vi "flow_to_coag_dose.vi"(4 "State":i16, 5 "Time":dbl format="%.2f", 6 "Sensor Values":dbl[](array[numeric]), 7 "Set Points":dbl[](array[numeric])) -> (0 "required data":T1={"Set Point names"=["pump flow (mL/s)", "", ""], "required number of setpoints"=1, "required number of sensors"=1, "Sensor names"=["raw flow rate (L/s)"]}, 3 "output value":dbl)   [LabVIEW 2019]
uses:
  Global Plantita Parameters.vi
panel:
  # "Enter the correct information for this control code in the required data structure below. Then make the current value default by right clicking on the border of the data structure. Select \"data operations\" and then select \"make current value default\". These values will be displayed by process controller."
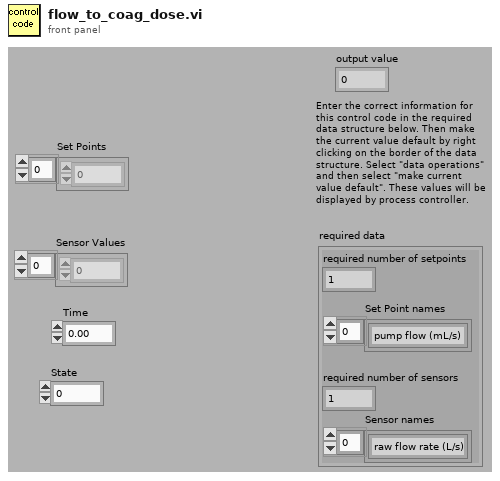
[diagram p1: front panel]
types:
  T1 = cluster{"Set Point names":string[], "required number of setpoints":u8, "required number of sensors":u8, "Sensor names":string[]}
  T2 = cluster{"flocculation_time(s)":dbl, "clarification_time(s)":dbl, "height_ff(m)":dbl, "C_coag_stock(g/L)":dbl}
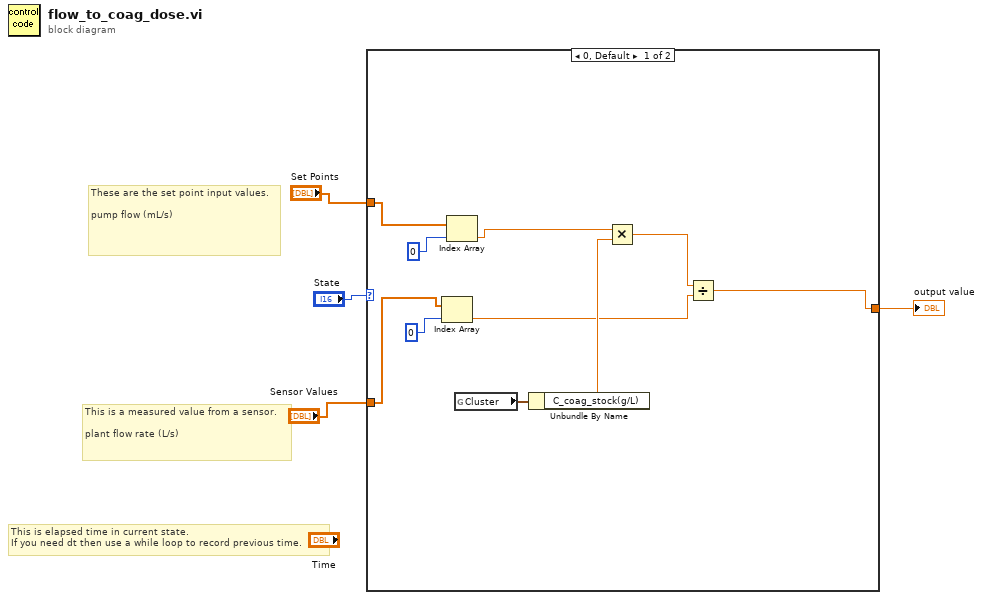
[diagram p0: block diagram]
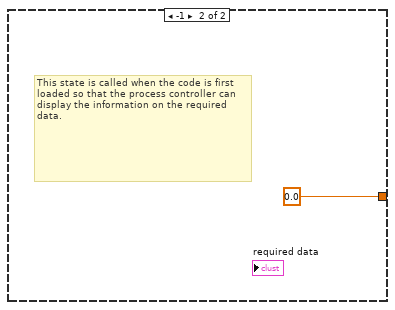
[diagram p2: hidden frame]
diagram:
  # "These are the set point input values.\n\npump flow (mL/s)"
  # "This is a measured value from a sensor.\n\nplant flow rate (L/s)"
  # "This is elapsed time in current state.\nIf you need dt then use a while loop to record previous time."
  n1 = case shown="0, Default" "State" {
    tunnel: [w11 0.0 ("fraction on")] -> w1
    tunnel: "Set Points" -> [w9 _]
    tunnel: "Sensor Values" -> [w7 _]
    frame 0, Default {
      n2 = Index Array(array=w7, index=0) -> (element=w5:dbl)
      n3 = Index Array(array=w9, index=0) -> (element=w8:dbl)
      n4 = global read "Global Plantita Parameters.vi" "Cluster"() -> (w14:T2)
      n5 = Unbundle By Name(w14) -> ("C_coag_stock(g/L)"=w13:dbl)
      n6 = Multiply(x=w8, y=w13) -> (x*y=w12:dbl)
      n7 = Divide(x=w12, y=w5) -> (x/y=w11:dbl)
    }
    frame -1 {
      # "This state is called when the code is first loaded so that the process controller can display the information on the required data."
    }
  }
  "output value" <- w1
